vi "Hitrap_DiagnosticBox.ProcPeriodic.vi"(0 "i ref in":refnum<vi>, 3 "ms timeout (10000)":i32=10000, 5 "error in (no error)":errorcluster) -> (14 "i ref out":refnum<vi>, 17 "timed out":bool, 19 "error out":errorcluster)   [LabVIEW 2014, in "Hitrap_DiagnosticBox.lvlib"]
doc: "This method serves to periodically do things like reading values from the HW. Methods that should be executed periodically should be called from THIS methode. Add code here."
uses:
  Hitrap_DiagnosticBox.lvlib
  CSMotion/NanotecSMCPD/NanotecSMCPD.lvlib
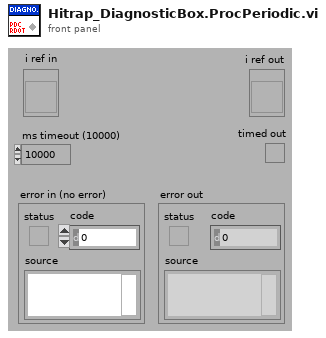
[diagram p1: front panel]
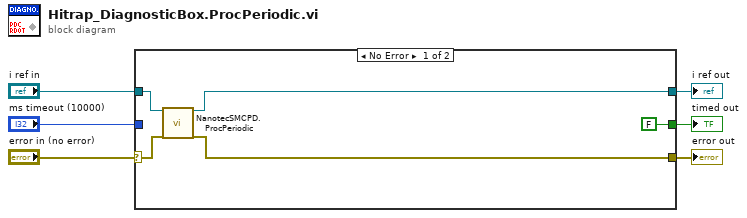
[diagram p0: block diagram]
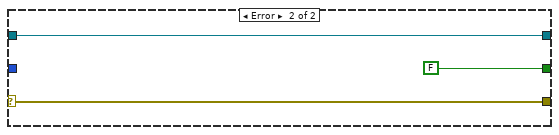
[diagram p2: hidden frame]
diagram:
  n1 = case shown="No Error" "error in (no error)" {
    selector: "error in (no error)" -> [w9 w13]
    tunnel: [w8 w13] -> w5
    tunnel: "i ref in" -> [w10 w14]
    tunnel: [w7 w14] -> w3
    tunnel: [FALSE FALSE] -> w2
    tunnel: "ms timeout (10000)" -> [_ _]
    frame No Error {
      n2 = call "NanotecSMCPD.ProcPeriodic.vi"("i ref in"=w10, "error in (no error)"=w9) -> ("i ref out"=w7:refnum<vi>, "error out"=w8:errorcluster)  [unwired: 15 in, 1 out]
    }
    frame Error {
    }
  }
  "error out" <- w5
  "i ref out" <- w3
  "timed out" <- w2
